vi "Read Data Type.vi"(8 "error in (no error)":errorcluster, 11 "Sender in":refnum<class "Sender.lvclass">) -> (0 "error out":errorcluster, 2 "Data Type":string(combo), 3 "Sender out":refnum<class "Sender.lvclass">)   [LabVIEW 2023, in "Sender.lvclass"]
uses:
  Sender.lvclass
  Sender.lvclass/Sender.ctl
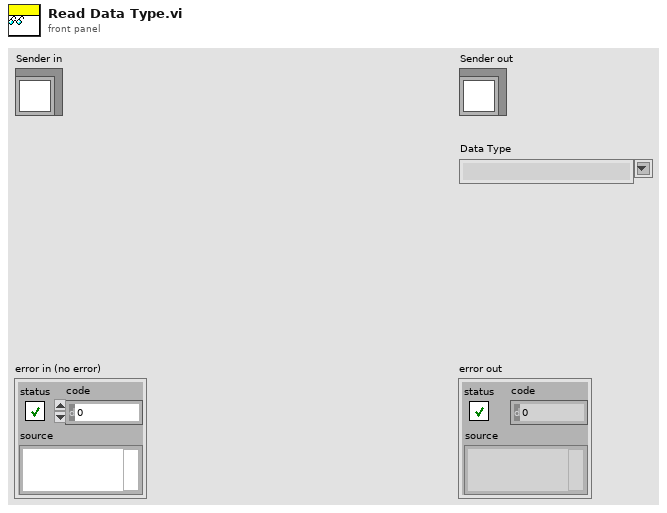
[diagram p1: front panel]
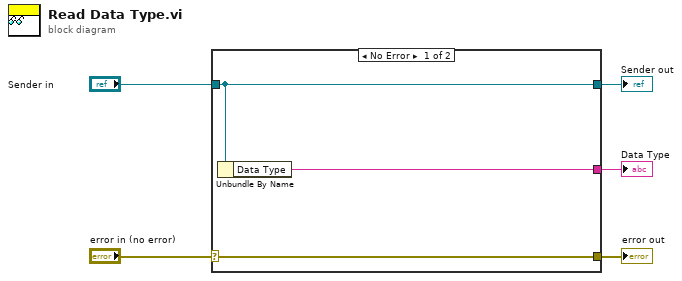
[diagram p0: block diagram]
diagram:
  n1 = case shown="No Error" "error in (no error)" {
    selector: "error in (no error)" -> [w8 w9]
    tunnel: [w8 w9] -> w4
    tunnel: [w7 w10] -> w2
    tunnel: "Sender in" -> [w7 w10]
    tunnel: [w6 _] -> w1
    frame No Error {
      n2 = Unbundle By Name(w7) -> ("Data Type"=w6:string)
    }
    frame Error {
    }
  }
  "error out" <- w4
  "Sender out" <- w2
  "Data Type" <- w1
